vi "Keithley2400_SR830_4Probe_Resistance_Measurement.vi"() -> ()   [LabVIEW 2018]
uses:
  <instrlib>/Stanford Research 830/Public/Data/Read (All Parameters).vi
  <instrlib>/Keithley 24XX/Public/Data/Read (Single Point).vi
  <instrlib>/Keithley 24XX/Keithley 24XX.lvlib
  <instrlib>/Stanford Research 830/Stanford Research 830.lvlib
panel:
  out "dup path":path
  in  "File Name":string
  in  "Data Save Path:":path
  in  "I_leak vs Vg":enum32{"XY Graph", "Waveform (Time)"}(tab)
  out "I_leak vs Vg : XYGraph":cluster{"Y":dbl[], "Y":dbl[]}[](graph)
  out "I_leak vs Vg : TimeGraph":cluster{dbl, "Current":sgl}[](graph)
  in  "Gate Voltage\nInitial (V)":dbl
  out "Gate Voltage\nTraversal Direction":enum16{"Upward", "Downward"}(ring)
  in  "Series Resistance \n(Apparatus Constant)":dbl
  in  "stop":bool
  out "Max/Min(-) \nGate Voltage (V)":dbl=80.0
  in  "Gate Voltage \nStep Size (V)":dbl
  in  "High Gate \nVoltage (V)":dbl
  in  "Low Gate \nVoltage (V)":dbl
  out "Compliance\n Level (A)":dbl=0.1
  in  "Theta vs Vg":enum32{"XY Graph", "Waveform (Time)"}(tab)
  out "Theta vs Vg : XYGraph":cluster{"Y":dbl[], "Y":dbl[]}[](graph)
  out "Theta vs Vg : TimeGraph":cluster{dbl, "Theta-Value":dbl}[](graph)
  in  "R vs Vg":enum32{"XY Graph", "Waveform (Time)"}(tab)
  out "Resistance vs Vg : XYGraph":cluster{"Y":dbl[], "Y":dbl[]}[](graph)
  out "R vs Vg : TimeGraph":cluster{dbl, dbl}[](graph)
  in  "Sensitivity (Initial Value)":i16(ring)=-1 items=["Auto Gain"=-1, "2 nV/fA"=0, "5 nV/fA"=1, "10 nV/fA"=2, "20 nV/fA"=3, "50 nV/fA"=4, "100 nV/fA"=5, "200 nV/fA"=6, "500 nV/fA"=7, "1 uV/pA"=8, "2 uV/pA"=9, "5 uV/pA"=10, "10 uV/pA"=11, "20 uV/pA"=12, "50 uV/pA"=13, "100 uV/pA"=14, "200 uV/pA"=15, "500 uV/pA"=16, "1 mV/nA"=17, "2 mV/nA"=18, "5 mV/nA"=19, "10 mV/nA"=20, "20 mV/nA"=21, "50 mV/nA"=22, "100 mV/nA"=23, "200 mV/nA"=24, "500 mV/mA"=25, "1 V/uA"=26]
  in  "Dynamic Reserve (-1 = Auto)":i16(ring)=-1 items=["Auto Reserve"=-1, "High Reserve"=0, "Normal"=1, "Low Noise"=2]
  in  "Input Connection (0: Single-Ended Voltage)":u16(ring) items=["Single-Ended Voltage", "Differential Voltage", "1 MOhm Current Gain", "100 MOhm Current Gain"]
  out "Input Coupling (0: AC)":u16(ring) items=["AC", "DC"]
  in  "Time Constant (8: 100ms)":u16(ring)=8 items=["10 us", "30 us", "100 us", "300 us", "1 ms", "3 ms", "10 ms", "30 ms", "100 ms", "300 ms", "1 s", "3 s", "10 s", "30 s", "100 s", "300 s", "1 ks", "3 ks", "10 ks", "30 ks"]
  in  "SR830 VISA resource name":refnum<visa-resource-name>
  in  "Trigger Source (0: Internal)":u16(ring) items=["Internal", "External"]
  out "Manual Phase (0 Degree)":dbl
  out "Detection Harmonic Number":dbl=1.0
  out "External Reference Trigger (0: Sine Zero Crossing)":u16(ring) items=["Sine Zero Crossing", "TTL Rising Edge", "TTL Falling Edge"]
  in  "Internal Reference Frequency (1000 Hz)":dbl=1000.0
  in  "Reference Source (1: Internal)":u16(ring)=1 items=["External", "Internal"]
  in  "Sine Output Amplitude (V)":dbl=1.0
  in  "Serial Configuration":T1={"Baud Rate"=9600, "Parity"=0, "Data Bits"=8, "Stop Bits"=10, "Flow Control"=0} {"Flow Control" items=["None", "XON/XOFF", "RTS/CTS", "XON/XOFF & RTS/CTS", "DTR/DSR", "XON/XOFF & DTR/DSR"]; "Stop Bits" items=["1.0"=10, "1.5"=15, "2.0"=20]; "Data Bits" items=["7"=7, "8"=8]; "Parity" items=["None", "Odd", "Even", "Mark", "Space"]; "Baud Rate" items=["300"=300, "600"=600, "1200"=1200, "2400"=2400, "4800"=4800, "9600"=9600, "19200"=19200]}
  in  "Keithley24XX VISA resource name":refnum<visa-resource-name> caption="Keithley 24XX VISA resource name"
  out "Interal Measurement Time":u32
  # "MAKE SURE THE SOURCE METER IS ON TO ENSURE NO UNINTENDED JUMPS. PROGRAM WILL KEEP SOURCE METER ON ONCE RUN."
  # "Keithley 2400 SourceMeter"
  # "SR830 Lock In Amplifier"
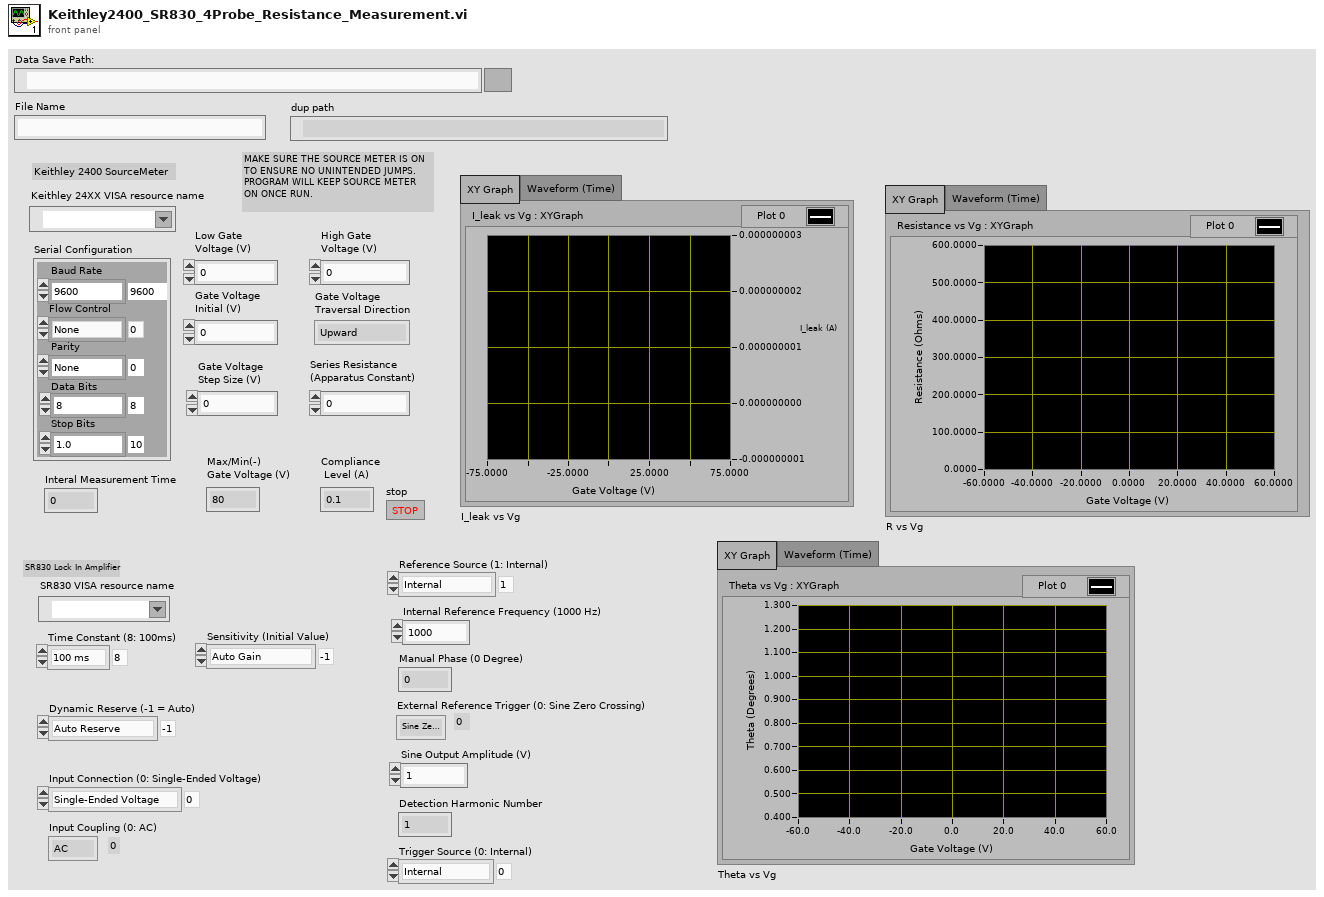
[diagram p1: front panel]
types:
  T1 = cluster{"Baud Rate":u32, "Parity":u16, "Data Bits":u16, "Stop Bits":u16, "Flow Control":u16}
  T2 = enum16{"open", "replace", "create", "open or create", "replace or create", "replace or create with confirmation"}
  T3 = cluster{"X-Value":dbl, "Y-Value":dbl, "R-Value":dbl, "Theta-Value":dbl, "Aux In 1 Value":dbl, "Aux In 2 Value":dbl, "Aux In 3 Value":dbl, "Aux In 4 Value":dbl, "Reference Frequency":dbl, "Channel 1 Display":dbl, "Channel 2 Display":dbl}
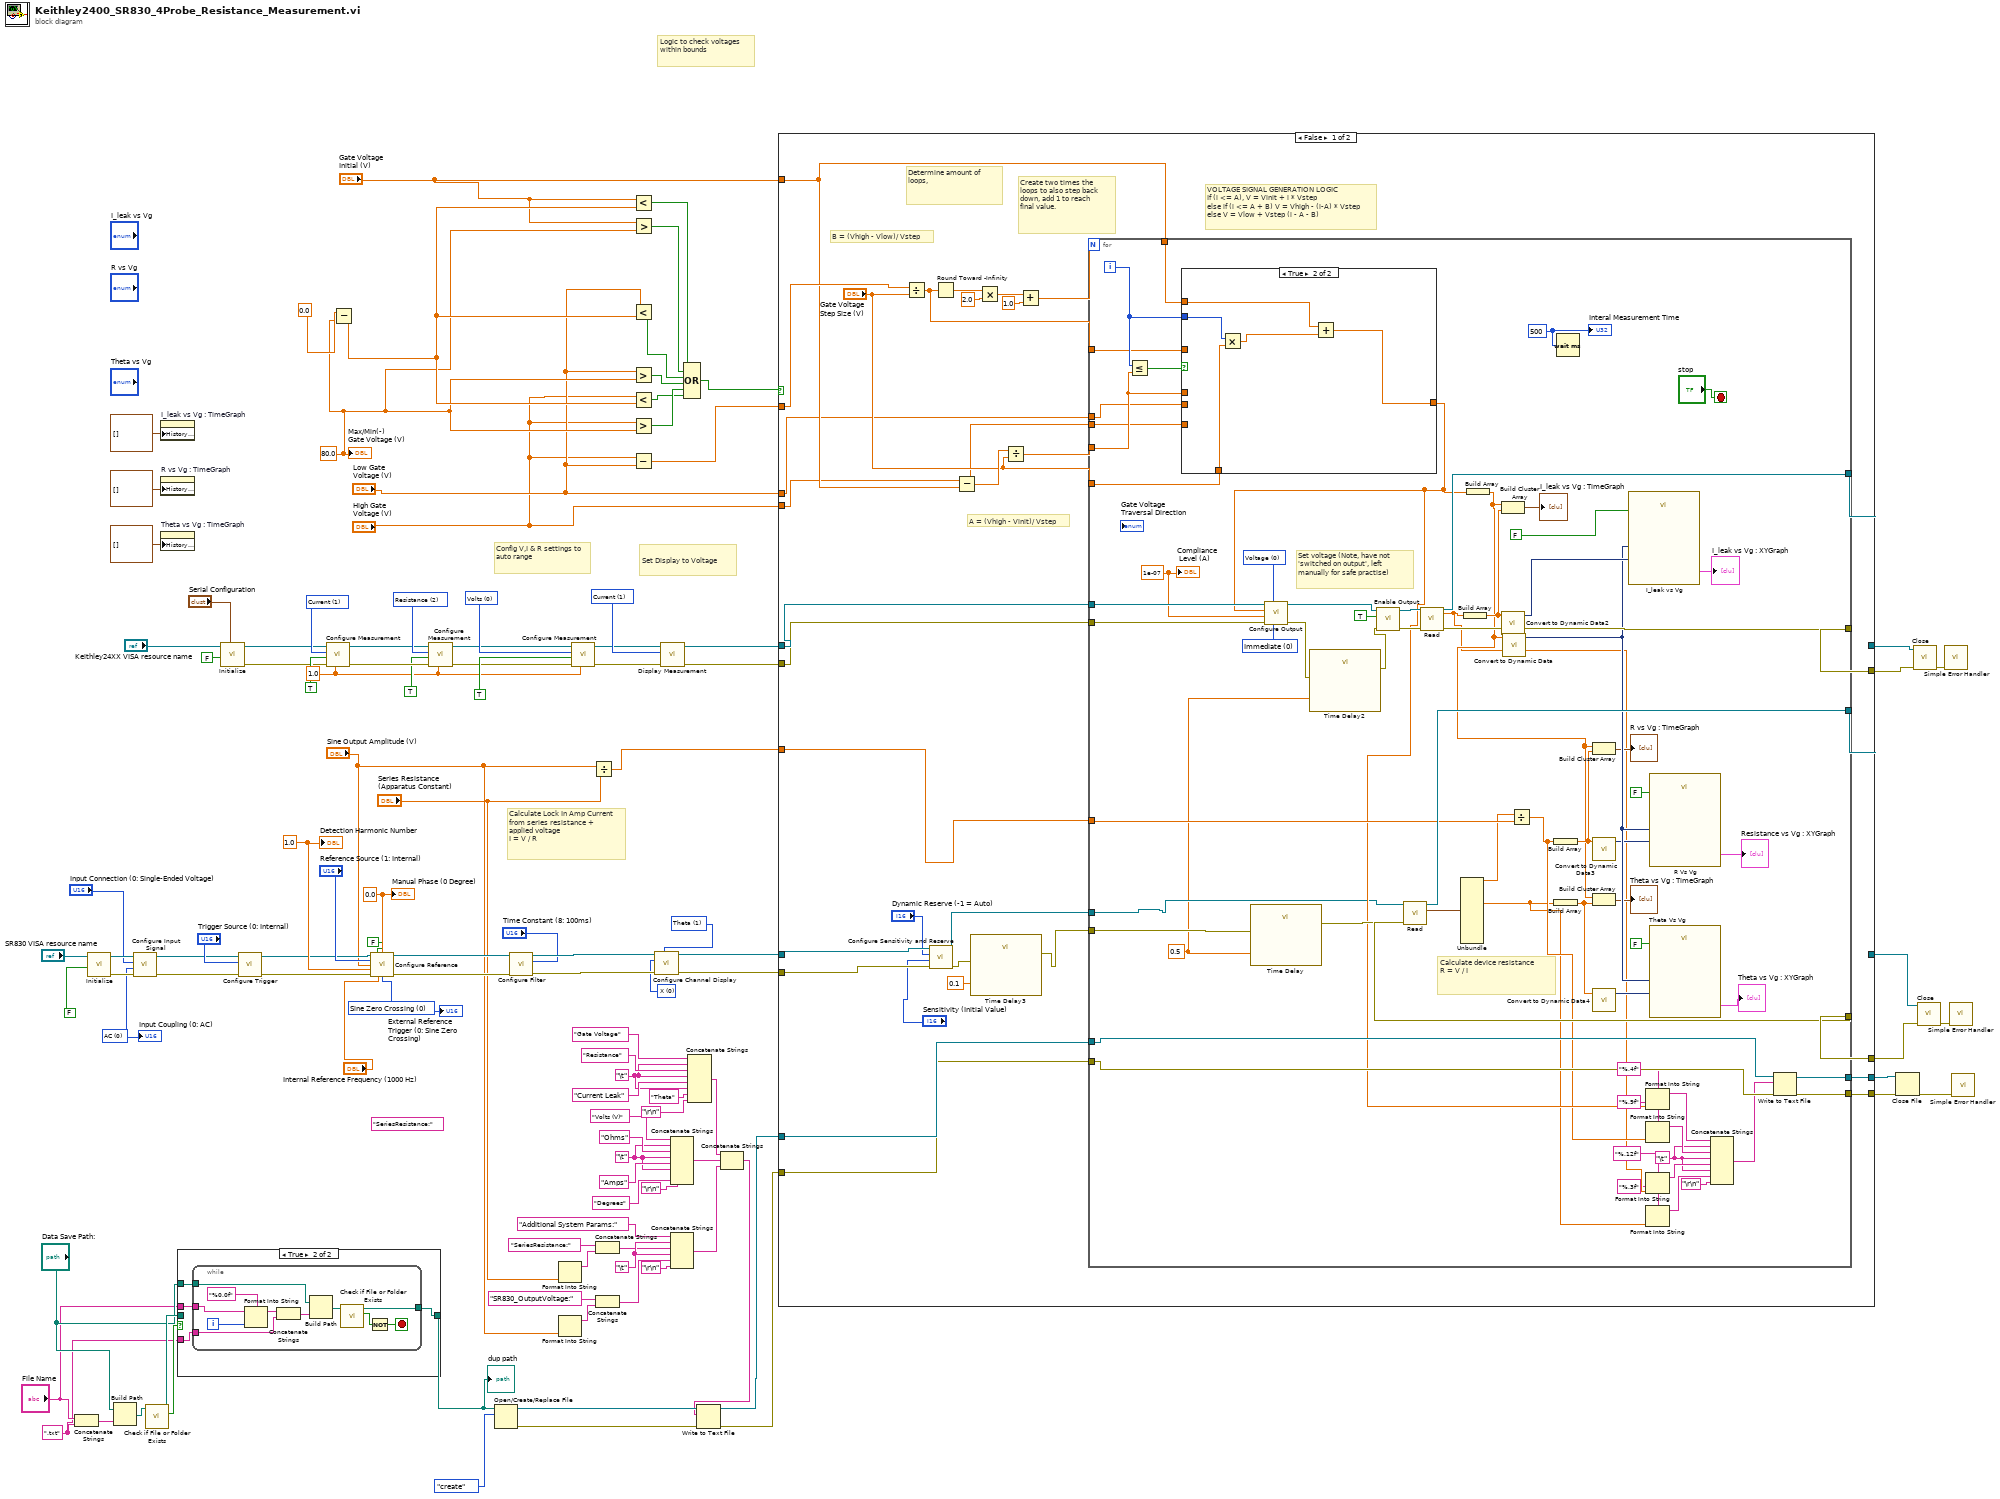
[diagram p0: block diagram]
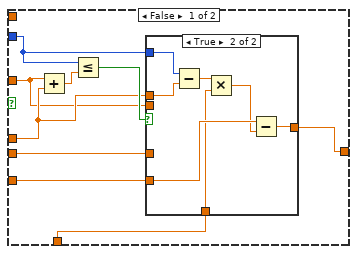
[diagram p3: hidden frame]
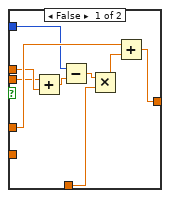
[diagram p4: hidden frame]
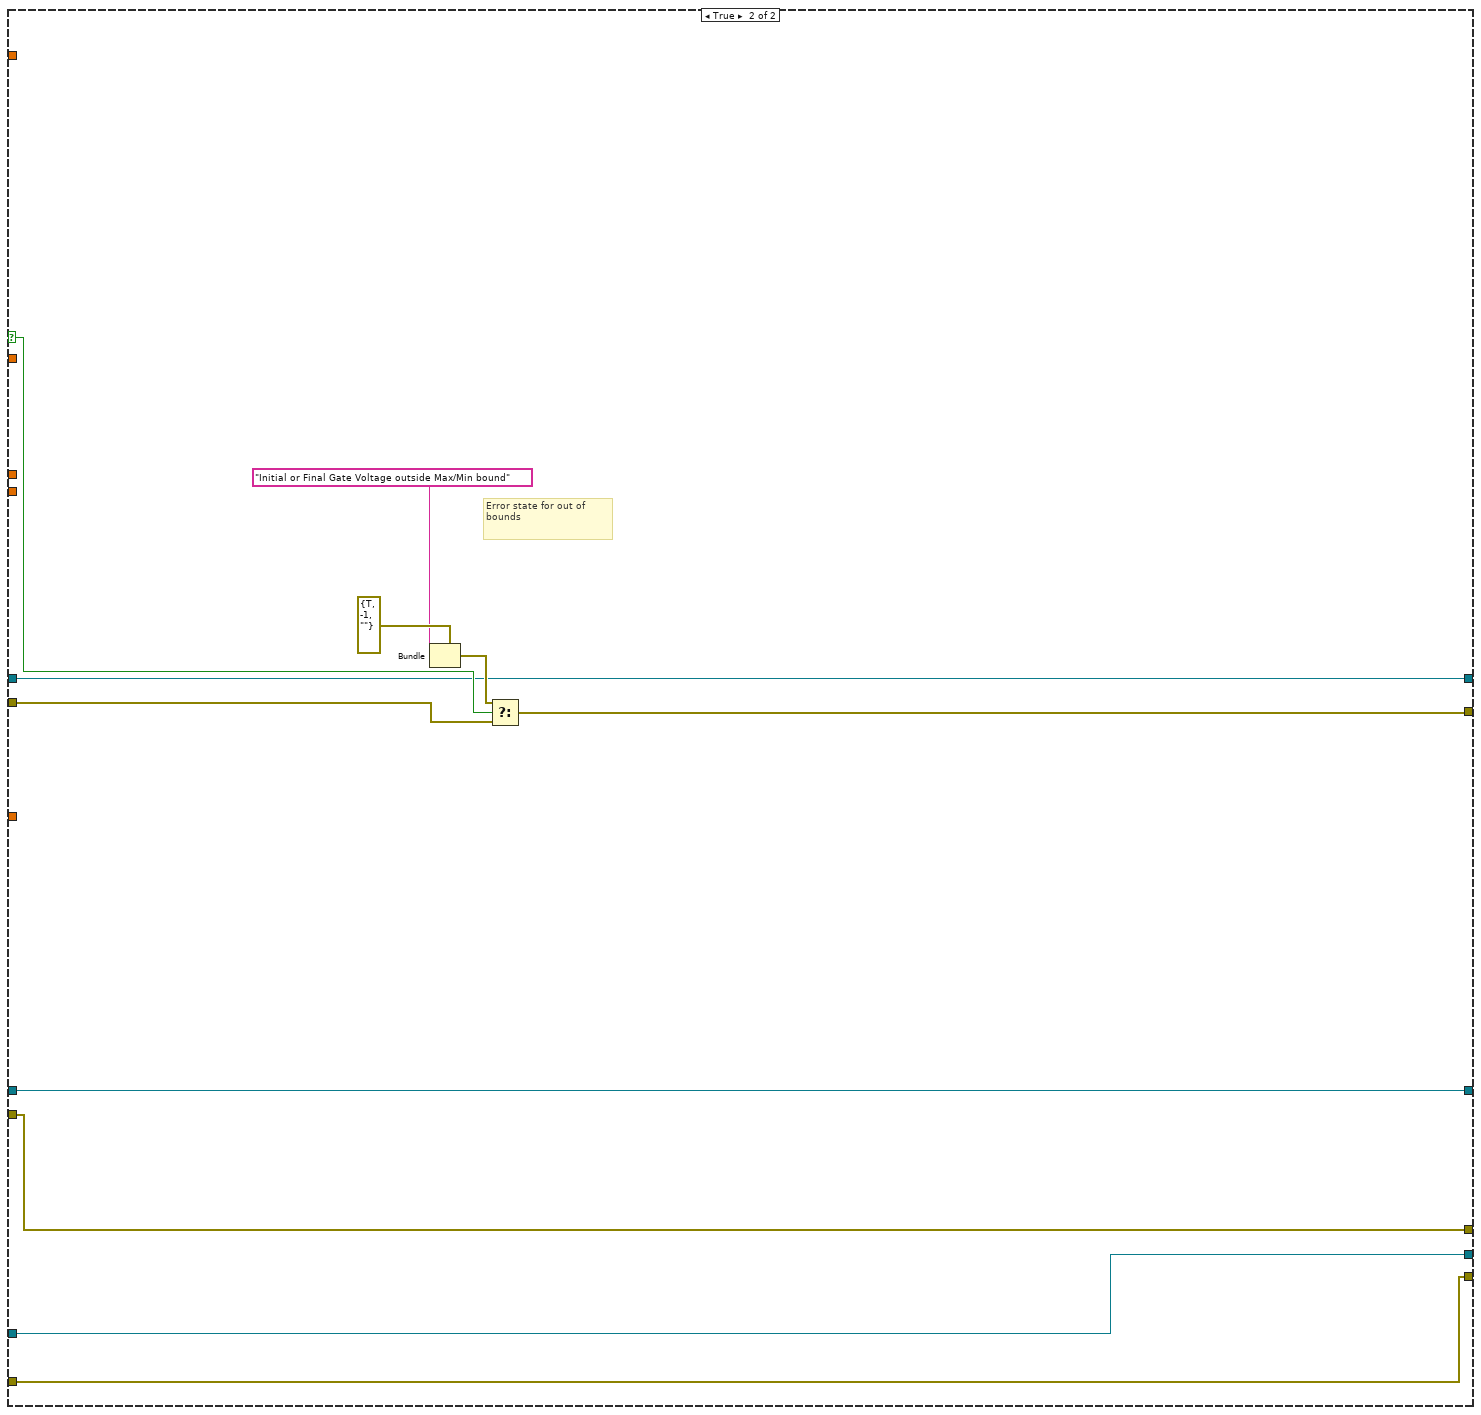
[diagram p5: hidden frame]
diagram:
  w5 = "\t"
  w9 = "\t"
  w14 = "\t"
  (unwired) "SeriesResistance:" ("string")
  w37 = ".txt"
  w44 = 1.0 ("Manual Range (1.0)")
  w71 = 0.0 ("Manual Phase (0 Degree)")
  w72 = 1.0 ("Detection Harmonic Number (1)")
  w73 = u16 0 items=["Sine Zero Crossing", "TTL Rising Edge", "TTL Falling Edge"] ("External Reference Trigger (0: Sine Zero Crossing)")
  w77 = u16 0 items=["AC", "DC"] ("Input Coupling (0: AC)")
  w59 = u16 0 items=["X", "R", "X Noise", "Aux In 1", "Aux In 2"] ("Channel 1 Display (0: X)")
  w87 = u16 1 items=["Y", "Theta", "Y Noise", "Aux In 3", "Aux In 4"] ("Channel 2 Display  (0: Y)")
  w94 = u16 1 items=["Voltage", "Current", "Resistance"] ("Displayed Measurement (0: Voltage)")
  w103 = u16 2 items=["Volts", "Current", "Resistance"] ("Function (0: Volts)")
  w107 = u16 1 items=["Volts", "Current", "Resistance"] ("Function (0: Volts)")
  w48 = 80.0
  w113 = u16 0 items=["Volts", "Current", "Resistance"] ("Function (0: Volts)")
  # "Logic to check voltages within bounds"
  # "Calculate Lock In Amp Current from series resistance + applied voltage\nI = V / R"
  # "Set Display to Voltage"
  # "Config V,I & R settings to auto range"
  n1 = Concatenate Strings("File Name", w37) -> (w43:string)
  n2 = call <instrlib>:"Initialize.vi"("Reset (True)"=FALSE, "VISA resource name"="SR830 VISA resource name") -> ("error out"=w84:errorcluster, "VISA resource name out"=w85:refnum<visa-resource-name>)  [unwired: 8 in]
  n3 = Build Path(base path="Data Save Path:", name or relative path=w43) -> (appended path=w42:path)
  n4 = call <instrlib>:"Configure Input Signal.vi"("error in (no error)"=w84, "Input Coupling (0: AC)"=w77, "Input Connection (0: Single-Ended Voltage)"="Input Connection (0: Single-Ended Voltage)", "VISA resource name"=w85) -> ("error out"=w68:errorcluster, "VISA resource name out"=w69:refnum<visa-resource-name>)  [unwired: 6 in]
  n5 = call <vilib>:"Check if File or Folder Exists.vi"("path"=w42) -> ("file or folder exists?"=w41:bool, "dup path"=w40:path)  [unwired: 8 in, 1 out]
  n6 = property on="I_leak vs Vg : TimeGraph" class="WFChart (strict)"("History Data"=cluster{dbl, "Current":sgl}[] []) -> ()  [unwired: 2 in, 2 out]
  n7 = property on="R vs Vg : TimeGraph" class="WFChart (strict)"("History Data"=cluster{dbl, dbl}[] []) -> ()  [unwired: 2 in, 2 out]
  n8 = property on="Theta vs Vg : TimeGraph" class="WFChart (strict)"("History Data"=cluster{dbl, "Theta-Value":dbl}[] []) -> ()  [unwired: 2 in, 2 out]
  n9 = case shown="True" w41 {
    tunnel: [w115 w116] -> w34
    tunnel: w40 -> [w115 _]
    tunnel: "Data Save Path:" -> [_ w117]
    tunnel: "File Name" -> [_ w119]
    tunnel: w37 -> [_ w118]
    frame False {
    }
    frame True {
      n10 = while {
        tunnel: w119 -> [w126]
        tunnel: w118 -> [w124]
        tunnel: w117 -> [w122]
        tunnel: [w120] -> w116
        i -> [w127]
        stop <- w129 stop-if-true
        n11 = Format Into String(format string="%0.0f", initial string=w126, w127) -> (resulting string=w125:string)  [unwired: 1 in, 1 out]
        n12 = Concatenate Strings(w125, w124) -> (w123:string)
        n13 = Build Path(base path=w122, name or relative path=w123) -> (appended path=w121:path)
        n14 = call <vilib>:"Check if File or Folder Exists.vi"("path"=w121) -> ("file or folder exists?"=w130:bool, "dup path"=w120:path)  [unwired: 8 in, 1 out]
        n15 = Not(x=w130) -> (.not. x?=w129:bool)
      }
    }
  }
  "dup path" <- w34
  n16 = call <instrlib>:"Initialize.vi"("Serial Configuration"="Serial Configuration", "Reset (True)"=FALSE, "VISA resource name"="Keithley24XX VISA resource name") -> ("error out"=w98:errorcluster, "VISA resource name out"=w99:refnum<visa-resource-name>)  [unwired: 7 in]
  n17 = call <instrlib>:"Configure Trigger.vi"("error in (no error)"=w68, "Trigger Source (0: Internal)"="Trigger Source (0: Internal)", "VISA resource name"=w69) -> ("error out"=w66:errorcluster, "VISA resource name out"=w67:refnum<visa-resource-name>)  [unwired: 7 in]
  n18 = call <instrlib>:"Configure Measurement.vi"("Manual Range (1.0)"=w44, "error in (no error)"=w98, "Enable Auto Range (T:Enable)"=TRUE, "Function (0: Volts)"=w107, "VISA resource name"=w99) -> ("error out"=w105:errorcluster, "VISA resource name out"=w100:refnum<visa-resource-name>)  [unwired: 5 in]
  n19 = Subtract(x=0.0, y=w48) -> (x-y=w53:dbl)
  n20 = call <instrlib>:"Configure Reference.vi"("VISA resource name"=w67, "Auto Phase (T: Enabled)"=FALSE, "Manual Phase (0 Degree)"=w71, "Reference Source (1: Internal)"="Reference Source (1: Internal)", "Sine Output Amplitude (1 V)"="Sine Output Amplitude (V)", "Detection Harmonic Number (1)"=w72, "error in (no error)"=w66, "Internal Reference Frequency (1000 Hz)"="Internal Reference Frequency (1000 Hz)", "External Reference Trigger (0: Sine Zero Crossing)"=w73) -> ("VISA resource name out"=w74:refnum<visa-resource-name>, "error out"=w75:errorcluster)  [unwired: 5 in]
  n21 = call <instrlib>:"Configure Measurement.vi"("Manual Range (1.0)"=w44, "error in (no error)"=w105, "Enable Auto Range (T:Enable)"=TRUE, "Function (0: Volts)"=w103, "VISA resource name"=w100) -> ("error out"=w102:errorcluster, "VISA resource name out"=w101:refnum<visa-resource-name>)  [unwired: 5 in]
  n22 = Open/Create/Replace File(file path (use dialog)=w34, operation (0:open)=T2."create") -> (refnum out=w35:refnum<file>, error out=w33:errorcluster)  [unwired: 4 in, 1 out]
  n23 = call <instrlib>:"Configure Filter.vi"("error in (no error)"=w75, "Time Constant (8: 100ms)"="Time Constant (8: 100ms)", "VISA resource name"=w74) -> ("error out"=w96:errorcluster, "VISA resource name out"=w95:refnum<visa-resource-name>)  [unwired: 7 in]
  n24 = Format Into String("Series Resistance \n(Apparatus Constant)") -> (resulting string=w27:string)  [unwired: 3 in, 1 out]
  n25 = Format Into String("Sine Output Amplitude (V)") -> (resulting string=w26:string)  [unwired: 3 in, 1 out]
  n26 = call <instrlib>:"Configure Measurement.vi"("Manual Range (1.0)"=w44, "error in (no error)"=w102, "Enable Auto Range (T:Enable)"=TRUE, "Function (0: Volts)"=w113, "VISA resource name"=w101) -> ("error out"=w92:errorcluster, "VISA resource name out"=w93:refnum<visa-resource-name>)  [unwired: 5 in]
  n27 = Divide(x="Sine Output Amplitude (V)", y="Series Resistance \n(Apparatus Constant)") -> (x/y=w65:dbl)
  n28 = Concatenate Strings("SeriesResistance:" ("string"), w27) -> (w4:string)
  n29 = Concatenate Strings("SR830_OutputVoltage:" ("string"), w26) -> (w3:string)
  n30 = Less?(x="Gate Voltage\nInitial (V)", y=w53) -> (x < y?=w51:bool)
  n31 = Less?(x="Low Gate \nVoltage (V)", y=w53) -> (x < y?=w57:bool)
  n32 = Greater?(x="Low Gate \nVoltage (V)", y=w48) -> (0:w56:bool)
  n33 = Less?(x="High Gate \nVoltage (V)", y=w53) -> (x < y?=w54:bool)
  n34 = Greater?(x="High Gate \nVoltage (V)", y=w48) -> (0:w55:bool)
  n35 = Subtract(x="High Gate \nVoltage (V)", y="Low Gate \nVoltage (V)") -> (x-y=w49:dbl)
  n36 = Greater?(x="Gate Voltage\nInitial (V)", y=w48) -> (0:w52:bool)
  n37 = call <instrlib>:"Configure Channel Display.vi"("Channel 2 Display  (0: Y)"=w87, "error in (no error)"=w96, "Channel 1 Display (0: X)"=w59, "VISA resource name"=w95) -> ("error out"=w82:errorcluster, "VISA resource name out"=w83:refnum<visa-resource-name>)  [unwired: 6 in]
  n38 = call <instrlib>:"Display Measurement.vi"("error in (no error)"=w92, "Displayed Measurement (0: Voltage)"=w94, "VISA resource name"=w93) -> ("error out"=w90:errorcluster, "VISA resource name out"=w91:refnum<visa-resource-name>)  [unwired: 7 in]
  n39 = Concatenate Strings("Volts (V)" ("string"), w9, "Ohms" ("string"), w9, "Amps" ("string"), w9, "Degrees" ("string"), "\r\n") -> (w20:string)
  n40 = Concatenate Strings("Additional System Params:" ("string"), w5, w4, w5, w3, "\r\n") -> (w6:string)
  n41 = Compound Arithmetic op=OR(w51, w52, w57, w56, w55, w54) -> (w50:bool)
  n42 = Concatenate Strings("Gate Voltage" ("string"), w14, "Resistance" ("string"), w14, "Current Leak" ("string"), w14, "Theta" ("string"), "\r\n") -> (w21:string)
  n43 = Concatenate Strings(w21, w20, w6) -> (w1:string)
  n44 = Write to Text File(file (use dialog)=w35, text=w1, error in=w33) -> (refnum out=w31:refnum<file>, error out=w30:errorcluster)  [unwired: 1 in, 1 out]
  n45 = case shown="False" w50 {
    selector: w50 -> [_ w271]
    tunnel: w90 -> [w161 w270]
    tunnel: w91 -> [w162 w265]
    tunnel: [w160 w265] -> w111
    tunnel: [w159 w266] -> w110
    tunnel: w83 -> [w154 w264]
    tunnel: w82 -> [w155 w263]
    tunnel: [w157 w264] -> w81
    tunnel: [w156 w263] -> w80
    tunnel: w65 -> [w151 _]
    tunnel: w49 -> [w146 _]
    tunnel: "Low Gate \nVoltage (V)" -> [w139 _]
    tunnel: "High Gate \nVoltage (V)" -> [w140 _]
    tunnel: "Gate Voltage\nInitial (V)" -> [w142 _]
    tunnel: w31 -> [w135 w262]
    tunnel: w30 -> [w134 w261]
    tunnel: [w133 w262] -> w29
    tunnel: [w132 w261] -> w28
    frame False {
      # "VOLTAGE SIGNAL GENERATION LOGIC\nIf (i <= A), V = Vinit + i * Vstep\nelse if (i <= A + B) V = Vhigh - (i-A) * Vstep\nelse V = Vlow + Vstep (i - A - B)"
      # "B = (Vhigh - Vlow)/ Vstep"
      # "A = (Vhigh - Vinit)/ Vstep"
      # "Create two times the loops to also step back down, add 1 to reach final value."
      # "Determine amount of loops,"
      n46 = Divide(x=w146, y="Gate Voltage \nStep Size (V)") -> (x/y=w141:dbl)
      n47 = call <instrlib>:"Configure Sensitivity and Reserve.vi"("error in (no error)"=w155, "Sensitivity (-1: Auto gain)"="Sensitivity (Initial Value)", "Dynamic Reserve (-1: Auto Reserve)"="Dynamic Reserve (-1 = Auto)", "VISA resource name"=w154) -> ("error out"=w137:errorcluster, "VISA resource name out"=w153:refnum<visa-resource-name>)  [unwired: 6 in]
      n48 = Round Toward -Infinity(1:w141) -> (0:w149:dbl)
      n49 = Subtract(x=w140, y=w142) -> (x-y=w145:dbl)
      n50 = call "Time Delay3"("error in (no error)"=w137, "Delay Time (s)"=0.1) -> ("error out"=w138:errorcluster)  [unwired: 9 in]
      n51 = Multiply(x=w149, y=2.0) -> (x*y=w148:dbl)
      n52 = Divide(x=w145, y="Gate Voltage \nStep Size (V)") -> (x/y=w143:dbl)
      n53 = Add(x=w148, y=1.0) -> (x+y=w147:dbl)
      n54 = for {
        N: w147 -> [_]
        tunnel: w162 -> [w226]
        tunnel: w161 -> [w187]
        tunnel: [w230] -> w160
        tunnel: [w229] -> w159
        tunnel: [w218] -> w157
        tunnel: [w219] -> w156
        tunnel: w153 -> [w164]
        tunnel: w138 -> [w165]
        tunnel: w151 -> [w216]
        tunnel: "Gate Voltage \nStep Size (V)" -> [w193]
        tunnel: w143 -> [w191]
        tunnel: w142 -> [w195]
        tunnel: w141 -> [w192]
        tunnel: w140 -> [w190]
        tunnel: w139 -> [w189]
        tunnel: w135 -> [w184]
        tunnel: w134 -> [w183]
        tunnel: [w182] -> w133
        tunnel: [w181] -> w132
        i -> [w194]
        stop <- "stop" stop-if-true
        w176 = "\t"
        w188 = u16 0 items=["Immediate", "Triggered"] ("Output Type  (0: Immediate)")
        w163 = 0.5 ("Delay Time (s)")
        w227 = u32 500 ("milliseconds to wait")
        w225 = 1e-07 ("Compliance  Level (0.1)")
        w221 = u16 0 items=["Voltage", "Current"] ("Source Mode  (0: Voltage)")
        # "Calculate device resistance\nR = V / I"
        # "Set voltage (Note, have not 'switched on output', left manually for safe practise)"
        n55 = Less Or Equal?(x=w194, y=w191) -> (x <= y?=w196:bool)
        n56 = case shown="True" w196 {
          tunnel: [w237 w256] -> w173
          tunnel: w195 -> [_ w259]
          tunnel: w194 -> [w234 w260]
          tunnel: w193 -> [w235 w257]
          tunnel: w192 -> [w231 _]
          tunnel: w191 -> [w233 _]
          tunnel: w190 -> [w236 _]
          tunnel: w189 -> [w232 _]
          frame False {
            n57 = Add(x=w231, y=w233) -> (x+y=w238:dbl)
            n58 = Less Or Equal?(x=w234, y=w238) -> (x <= y?=w239:bool)
            n59 = case shown="True" w239 {
              tunnel: [w245 w254] -> w237
              tunnel: w236 -> [_ w255]
              tunnel: w235 -> [w247 w252]
              tunnel: w234 -> [w242 w251]
              tunnel: w233 -> [w241 w250]
              tunnel: w232 -> [w248 _]
              tunnel: w231 -> [w240 _]
              frame False {
                n60 = Add(x=w240, y=w241) -> (x+y=w243:dbl)
                n61 = Subtract(x=w242, y=w243) -> (x-y=w244:dbl)
                n62 = Multiply(x=w244, y=w247) -> (x*y=w246:dbl)
                n63 = Add(x=w248, y=w246) -> (x+y=w245:dbl)
              }
              frame True {
                n64 = Subtract(x=w251, y=w250) -> (x-y=w253:dbl)
                n65 = Multiply(x=w253, y=w252) -> (x*y=w249:dbl)
                n66 = Subtract(x=w255, y=w249) -> (x-y=w254:dbl)
              }
            }
          }
          frame True {
            n67 = Multiply(x=w260, y=w257) -> (x*y=w258:dbl)
            n68 = Add(x=w259, y=w258) -> (x+y=w256:dbl)
          }
        }
        n69 = call "Time Delay"("error in (no error)"=w165, "Delay Time (s)"=w163) -> ("error out"=w214:errorcluster)  [unwired: 9 in]
        n70 = call <instrlib>:"Configure Output.vi"("Output Type  (0: Immediate)"=w188, "Source Mode  (0: Voltage)"=w221, "error in (no error)"=w187, "Compliance  Level (0.1)"=w225, "Output Level (0)"=w173, "VISA resource name"=w226) -> ("error out"=w186:errorcluster, "VISA resource name out"=w224:refnum<visa-resource-name>)  [unwired: 4 in]
        n71 = call "Time Delay2"("error in (no error)"=w186, "Delay Time (s)"=w163) -> ("error out"=w185:errorcluster)  [unwired: 9 in]
        n72 = call <instrlib>:"Enable Output.vi"("error in (no error)"=w185, "Enable Output (T: Enable)"=TRUE, "VISA resource name"=w224) -> ("error out"=w223:errorcluster, "VISA resource name out"=w222:refnum<visa-resource-name>)  [unwired: 7 in]
        n73 = call-poly <instrlib>:"Read.vi"("error in (no error)"=w214, "VISA resource name"=w164) -> ("error out"=w219:errorcluster, "Parameter Values"=w217:T3, "VISA resource name out"=w218:refnum<visa-resource-name>)  [unwired: 7 in]
        n74 = call-poly <instrlib>:"Read.vi"("VISA resource name"=w222, "error in (no error)"=w223) -> ("VISA resource name out"=w230:refnum<visa-resource-name>, "Current"=w170:sgl, "error out"=w229:errorcluster)  [unwired: 7 in, 4 out]
        n75 = Unbundle(w217) -> ("X-Value"=w215:dbl, "Theta-Value"=w171:dbl)  [unwired: 9 out]
        n76 = Build Array(w170) -> (w211:sgl[])
        n77 = Build Array(w173) -> (w197:dbl[])
        n78 = Build Cluster Array(w197, w211) -> (→"I_leak vs Vg : TimeGraph":cluster{dbl, "Current":sgl}[])
        n79 = call "Convert to Dynamic Data2"("Array"=w211) -> ("Dynamic Data Type"=w210:dynamicdata)  [unwired: 3 in]
        n80 = call "Convert to Dynamic Data"("Array"=w197) -> ("Dynamic Data Type"=w209:dynamicdata)  [unwired: 3 in]
        n81 = Divide(x=w215, y=w216) -> (x/y=w172:dbl)
        n82 = Build Array(w172) -> (w208:dbl[])
        n83 = Build Array(w171) -> (w206:dbl[])
        n84 = Wait (ms)(milliseconds to wait=w227) -> ()  [unwired: 1 out]
        n85 = Build Cluster Array(w197, w208) -> (→"R vs Vg : TimeGraph":cluster{dbl, dbl}[])
        n86 = call "Convert to Dynamic Data3"("Array"=w208) -> ("Dynamic Data Type"=w207:dynamicdata)  [unwired: 3 in]
        n87 = Build Cluster Array(w197, w206) -> (→"Theta vs Vg : TimeGraph":cluster{dbl, "Theta-Value":dbl}[])
        n88 = call "Convert to Dynamic Data4"("Array"=w206) -> ("Dynamic Data Type"=w205:dynamicdata)  [unwired: 3 in]
        n89 = call "I_leak vs Vg"("Reset"=FALSE, "Y Input"=w210, "X Input"=w209) -> ("XY Graph"=→"I_leak vs Vg : XYGraph":cluster{"X":dbl[], "Y":dbl[]}[])  [unwired: 7 in, 1 out]
        n90 = Format Into String(format string="%.4f", w173) -> (resulting string=w180:string)  [unwired: 2 in, 1 out]
        n91 = Format Into String(format string="%.9f", w172) -> (resulting string=w179:string)  [unwired: 2 in, 1 out]
        n92 = Format Into String(format string="%.12f", w170) -> (resulting string=w178:string)  [unwired: 2 in, 1 out]
        n93 = Format Into String(format string="%.3f", w171) -> (resulting string=w177:string)  [unwired: 2 in, 1 out]
        n94 = call "R Vs Vg"("Reset"=FALSE, "Y Input"=w207, "X Input"=w209) -> ("XY Graph"=→"Resistance vs Vg : XYGraph":cluster{"X":dbl[], "Y":dbl[]}[])  [unwired: 7 in, 1 out]
        n95 = call "Theta Vs Vg"("Reset"=FALSE, "Y Input"=w205, "X Input"=w209) -> ("XY Graph"=→"Theta vs Vg : XYGraph":cluster{"X":dbl[], "Y":dbl[]}[])  [unwired: 7 in, 1 out]
        n96 = Concatenate Strings(w180, w176, w179, w176, w178, w176, w177, "\r\n") -> (w174:string)
        n97 = Write to Text File(file (use dialog)=w184, text=w174, error in=w183) -> (refnum out=w182:refnum<file>, error out=w181:errorcluster)  [unwired: 1 in, 1 out]
        "Compliance\n Level (A)" <- w225
        "Interal Measurement Time" <- w227
      }
    }
    frame True {
      # "Error state for out of bounds"
      n98 = Bundle(cluster=errorcluster {"status"=TRUE, "code"=-1, "source"=""} ("error constant"), "source"="Initial or Final Gate Voltage outside Max/Min bound") -> (w267:errorcluster)  [unwired: 2 in]
      n99 = Select(t=w267, s=w271, f=w270) -> (s? t:f=w266:errorcluster)
    }
  }
  n100 = Close File(refnum=w29, error in=w28) -> (error out=w32:errorcluster)  [unwired: 1 out]
  n101 = call <instrlib>:"Close.vi"("error in (no error)"=w110, "VISA resource name"=w111) -> ("error out"=w109:errorcluster)  [unwired: 9 in]
  n102 = call <instrlib>:"Close.vi"("error in (no error)"=w80, "VISA resource name"=w81) -> ("error out"=w97:errorcluster)  [unwired: 9 in]
  n103 = call <vilib>:"Simple Error Handler.vi"("error in (no error)"=w109) -> ()  [unwired: 4 in, 5 out]
  n104 = call <vilib>:"Simple Error Handler.vi"("error in (no error)"=w97) -> ()  [unwired: 4 in, 5 out]
  n105 = call <vilib>:"Simple Error Handler.vi"("error in (no error)"=w32) -> ()  [unwired: 4 in, 5 out]
  "Max/Min(-) \nGate Voltage (V)" <- w48
  "Input Coupling (0: AC)" <- w77
  "External Reference Trigger (0: Sine Zero Crossing)" <- w73
  "Detection Harmonic Number" <- w72
  "Manual Phase (0 Degree)" <- w71
